vi "ProjectOpenReferences.vi"(0 "Gateway IP Address (\"\": localhost)":string, 11 "error in (no error)":errorcluster) -> (4 "WorkspaceManager":T3, 6 "ModelManager":T1, 8 "ChannelFault":T2, 15 "error out":errorcluster)   [LabVIEW 2015, in "MiscHelperVIs.lvlib"]
uses:
  MiscHelperVIs.lvlib
  <vilib>/NI Veristand/Execution/Workspace/WorkspaceAPI.ctl
  NationalInstruments.VeriStand.ClientAPI
  <vilib>/NI Veristand/Execution/ChannelFaultManager/ChannelFaultAPI.ctl
  <vilib>/NI Veristand/Execution/ModelManager/ModelManagerAPI.ctl
  <vilib>/NI Veristand/Execution/Workspace/NI_VS Workspace ExecutionAPI.lvlib
  <vilib>/NI Veristand/Execution/ChannelFaultManager/NI_VS ChannelFault ExecutionAPI.lvlib
  <vilib>/NI Veristand/Execution/ModelManager/NI_VS ModelManager ExecutionAPI.lvlib
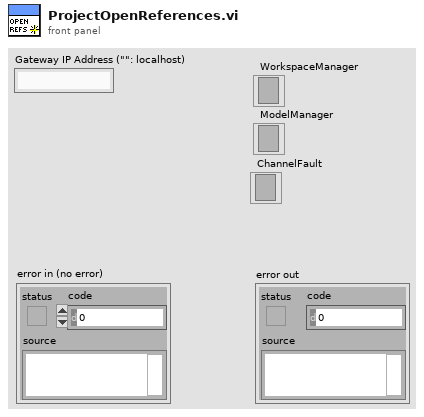
[diagram p1: front panel]
types:
  T1 = typedef "NI_VS ModelManager ExecutionAPI.lvlib/ModelManagerAPI.ctl" = refnum<k24>
  T2 = typedef "NI_VS ChannelFault ExecutionAPI.lvlib/ChannelFaultAPI.ctl" = refnum<k24>
  T3 = typedef "NI_VS Workspace ExecutionAPI.lvlib/WorkspaceAPI.ctl" = refnum<k24>
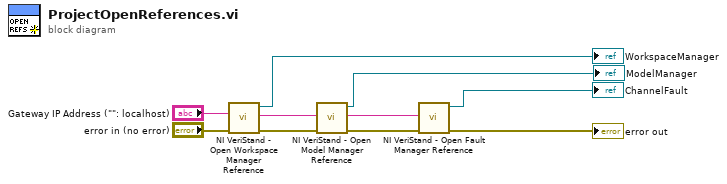
[diagram p0: block diagram]
diagram:
  n1 = call <vilib>:"NI VeriStand - Open Workspace Manager Reference.vi"("error in (no error)"="error in (no error)", "Gateway IP Address (\"\": localhost)"="Gateway IP Address (\"\": localhost)") -> ("error out"=w4:errorcluster, "WorkspaceManager"=→"WorkspaceManager":T3)  [unwired: 8 in]
  n2 = call <vilib>:"NI VeriStand - Open Model Manager Reference.vi"("error in (no error)"=w4, "Gateway IP Address (\"\": localhost)"="Gateway IP Address (\"\": localhost)") -> ("error out"=w1:errorcluster, "ModelManager"=→"ModelManager":T1)  [unwired: 8 in]
  n3 = call <vilib>:"NI VeriStand - Open Fault Manager Reference.vi"("error in (no error)"=w1, "Gateway IP Address (\"\": localhost)"="Gateway IP Address (\"\": localhost)") -> ("error out"=→"error out":errorcluster, "ChannelFault"=→"ChannelFault":T2)  [unwired: 8 in]
